vi "Realsense Cam Color Stream Start.vi"(8 "error in (no error)":errorcluster, 11 "Realsense Cam in":refnum<class "Realsense Cam.lvclass">) -> (0 "error out":errorcluster, 3 "Realsense Cam out":refnum<class "Realsense Cam.lvclass">)   [LabVIEW 2018]
uses:
  Realsense Cam.lvclass
  Private/Stream Types Enum STYP.ctl
  Private/Stream STYP.ctl
  Private/Activated Stream STYP.ctl
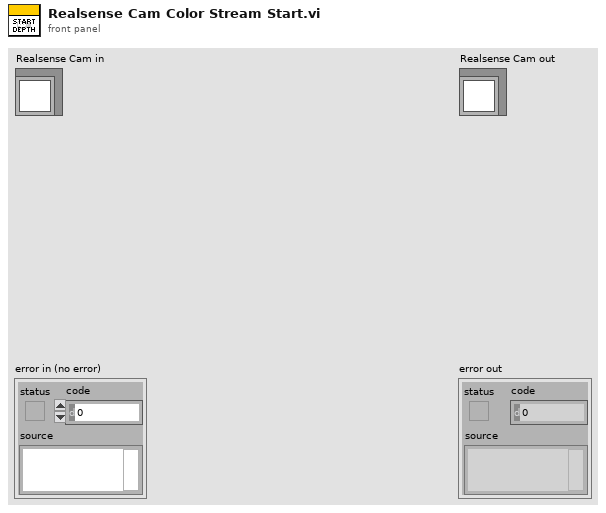
[diagram p1: front panel]
types:
  T1 = typedef "Realsense Cam.lvclass/Activated Stream STYP.ctl" = cluster{"Stream Type":T2, "Resolution":u16, "Profile Handle":u64, "Stream":T3}
  T2 = typedef "Realsense Cam.lvclass/Stream Types Enum STYP.ctl" = enum16{"Depth", "Left IR", "Right IR", "Color", "RGB Ext.", "Left IR Unrectified", "Right IR Unrectified"}
  T3 = typedef "Realsense Cam.lvclass/Stream STYP.ctl" = cluster{"Strings":string[], "Intrinsics":cluster{"width":i32, "height":i32, "fps":i32, "Profile":u64, "ppx":sgl, "ppy":sgl, "fx":sgl, "fy":sgl, "model":u32}[]}
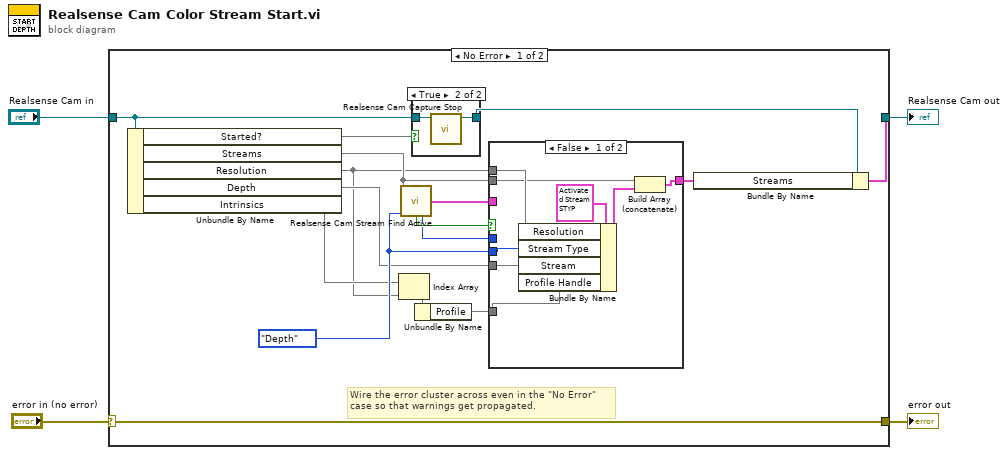
[diagram p0: block diagram]
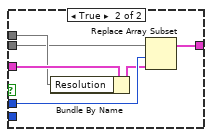
[diagram p2: hidden frame]
diagram:
  n1 = case shown="No Error" "error in (no error)" {
    selector: "error in (no error)" -> [w20 w39]
    tunnel: [w20 w39] -> w3
    tunnel: [w5 w38] -> w1
    tunnel: "Realsense Cam in" -> [w19 w38]
    frame No Error {
      w13 = Stream_Types_Enum_STYP."Depth" ("Stream Types")
      # "Wire the error cluster across even in the \"No Error\"\ncase so that warnings get propagated."
      n2 = Unbundle By Name(w19) -> ("Started?"=w18, "Streams"=w14, "Resolution"=w10, "Depth"=w12, "Intrinsics"=w11)
      n3 = Index Array(array=w11, index=w10) -> (element=w9)
      n4 = call "Realsense Cam Stream Find Active.vi"("Streams"=w14, "Stream Types"=w13) -> ("Activated Stream"=w15:T1, "Found?"=w17:bool, "Index"=w16:i32)  [unwired: 11 in]
      n5 = case shown="True" w18 {
        tunnel: w19 -> [w35 w37]
        tunnel: [w35 w36] -> w7
        frame False {
        }
        frame True {
          n6 = call-dynamic "Realsense Cam Capture Stop.vi"("Realsense Cam in"=w37) -> ("Realsense Cam out"=w36:refnum<class "Realsense Cam.lvclass">)  [unwired: 8 in, 2 out]
        }
      }
      n7 = Unbundle By Name(w9) -> ("Profile"=w8)
      n8 = case shown="False" w17 {
        tunnel: w16 -> [_ w31]
        tunnel: w15 -> [_ w34]
        tunnel: w10 -> [w24 w33]
        tunnel: w14 -> [w23 w32]
        tunnel: w13 -> [w25 _]
        tunnel: [w21 w29] -> w6
        tunnel: w12 -> [w26 _]
        tunnel: w8 -> [w27 _]
        frame False {
          n9 = Bundle By Name(cluster=T1 {"Stream Type"=enum."Color", "Resolution"=17, "Profile Handle"=0, "Stream"={"Strings"=["424 x 240 @6fps", "424 x 240 @15fps", "424 x 240 @30fps", "424 x 240 @60fps", "424 x 240 @90fps", "480 x 270 @6fps", "480 x 270 @15fps", "480 x 270 @30fps", "480 x 270 @60fps", "480 x 270 @90fps", "640 x 360 @6fps", "640 x 360 @15fps", "640 x 360 @30fps", "640 x 360 @60fps", "640 x 360 @90fps", "640 x 480 @6fps", "640 x 480 @15fps", "640 x 480 @30fps", "640 x 480 @60fps", "640 x 480 @90fps", "848 x 480 @6fps", "848 x 480 @15fps", "848 x 480 @30fps", "848 x 480 @60fps", "848 x 480 @90fps", "1280 x 720 @6fps", "1280 x 720 @15fps", "1280 x 720 @30fps", "1920 x 1080 @15fps", "1920 x 1080 @25fps"], "Intrinsics"=[{"width"=424, "height"=240, "fps"=6, "Profile"=521311384, "ppx"=210.19093, "ppy"=123.56658, "fx"=317.53546, "fy"=317.53546, "model"=4}, {"width"=424, "height"=240, "fps"=15, "Profile"=521310104, "ppx"=210.19093, "ppy"=123.56658, "fx"=317.53546, "fy"=317.53546, "model"=4}, {"width"=424, "height"=240, "fps"=30, "Profile"=521314712, "ppx"=210.19093, "ppy"=123.56658, "fx"=317.53546, "fy"=317.53546, "model"=4}, {"width"=424, "height"=240, "fps"=60, "Profile"=521313688, "ppx"=210.19093, "ppy"=123.56658, "fx"=317.53546, "fy"=317.53546, "model"=4}, {"width"=424, "height"=240, "fps"=90, "Profile"=521315736, "ppx"=210.19093, "ppy"=123.56658, "fx"=317.53546, "fy"=317.53546, "model"=4}, {"width"=480, "height"=270, "fps"=6, "Profile"=521314968, "ppx"=237.96481, "ppy"=139.0124, "fx"=357.2274, "fy"=357.2274, "model"=4}, {"width"=480, "height"=270, "fps"=15, "Profile"=521318808, "ppx"=237.96481, "ppy"=139.0124, "fx"=357.2274, "fy"=357.2274, "model"=4}, {"width"=480, "height"=270, "fps"=30, "Profile"=521316504, "ppx"=237.96481, "ppy"=139.0124, "fx"=357.2274, "fy"=357.2274, "model"=4}, {"width"=480, "height"=270, "fps"=60, "Profile"=521322904, "ppx"=237.96481, "ppy"=139.0124, "fx"=357.2274, "fy"=357.2274, "model"=4}, {"width"=480, "height"=270, "fps"=90, "Profile"=521312152, "ppx"=237.96481, "ppy"=139.0124, "fx"=357.2274, "fy"=357.2274, "model"=4}, {"width"=640, "height"=360, "fps"=6, "Profile"=521314200, "ppx"=317.2864, "ppy"=185.34987, "fx"=476.3032, "fy"=476.3032, "model"=4}, {"width"=640, "height"=360, "fps"=15, "Profile"=521319320, "ppx"=317.2864, "ppy"=185.34987, "fx"=476.3032, "fy"=476.3032, "model"=4}, {"width"=640, "height"=360, "fps"=30, "Profile"=521319064, "ppx"=317.2864, "ppy"=185.34987, "fx"=476.3032, "fy"=476.3032, "model"=4}, {"width"=640, "height"=360, "fps"=60, "Profile"=521321112, "ppx"=317.2864, "ppy"=185.34987, "fx"=476.3032, "fy"=476.3032, "model"=4}, {"width"=640, "height"=360, "fps"=90, "Profile"=521318296, "ppx"=317.2864, "ppy"=185.34987, "fx"=476.3032, "fy"=476.3032, "model"=4}, {"width"=640, "height"=480, "fps"=6, "Profile"=521313176, "ppx"=316.38187, "ppy"=247.13316, "fx"=635.0709, "fy"=635.0709, "model"=4}, {"width"=640, "height"=480, "fps"=15, "Profile"=521321368, "ppx"=316.38187, "ppy"=247.13316, "fx"=635.0709, "fy"=635.0709, "model"=4}, {"width"=640, "height"=480, "fps"=30, "Profile"=521309592, "ppx"=316.38187, "ppy"=247.13316, "fx"=635.0709, "fy"=635.0709, "model"=4}, {"width"=640, "height"=480, "fps"=60, "Profile"=521320088, "ppx"=316.38187, "ppy"=247.13316, "fx"=635.0709, "fy"=635.0709, "model"=4}, {"width"=640, "height"=480, "fps"=90, "Profile"=521322648, "ppx"=316.38187, "ppy"=247.13316, "fx"=635.0709, "fy"=635.0709, "model"=4}, {"width"=848, "height"=480, "fps"=6, "Profile"=521315992, "ppx"=420.38187, "ppy"=247.13316, "fx"=635.0709, "fy"=635.0709, "model"=4}, {"width"=848, "height"=480, "fps"=15, "Profile"=521317272, "ppx"=420.38187, "ppy"=247.13316, "fx"=635.0709, "fy"=635.0709, "model"=4}, {"width"=848, "height"=480, "fps"=30, "Profile"=521310616, "ppx"=420.38187, "ppy"=247.13316, "fx"=635.0709, "fy"=635.0709, "model"=4}, {"width"=848, "height"=480, "fps"=60, "Profile"=521310360, "ppx"=420.38187, "ppy"=247.13316, "fx"=635.0709, "fy"=635.0709, "model"=4}, {"width"=848, "height"=480, "fps"=90, "Profile"=521306776, "ppx"=420.38187, "ppy"=247.13316, "fx"=635.0709, "fy"=635.0709, "model"=4}, {"width"=1280, "height"=720, "fps"=6, "Profile"=521320600, "ppx"=634.5728, "ppy"=370.69974, "fx"=952.6064, "fy"=952.6064, "model"=4}, {"width"=1280, "height"=720, "fps"=15, "Profile"=521310872, "ppx"=634.5728, "ppy"=370.69974, "fx"=952.6064, "fy"=952.6064, "model"=4}, {"width"=1280, "height"=720, "fps"=30, "Profile"=521320344, "ppx"=634.5728, "ppy"=370.69974, "fx"=952.6064, "fy"=952.6064, "model"=4}, {"width"=1920, "height"=1080, "fps"=15, "Profile"=521627576, "ppx"=951.85925, "ppy"=556.0496, "fx"=1428.9095, "fy"=1428.9095, "model"=4}, {"width"=1920, "height"=1080, "fps"=25, "Profile"=521617080, "ppx"=951.85925, "ppy"=556.0496, "fx"=1428.9095, "fy"=1428.9095, "model"=4}]}} ("Activated Stream"), "Resolution"=w24, "Stream Type"=w25, "Stream"=w26, "Profile Handle"=w27) -> (w22:T1)
          n10 = Build Array (concatenate)(w23, w22) -> (w21:T1[])
        }
        frame True {
          n11 = Bundle By Name(cluster=w34, "Resolution"=w33) -> (w30:T1)
          n12 = Replace Array Subset(array=w32, new element=w30, index=w31) -> (w29:T1[])
        }
      }
      n13 = Bundle By Name(cluster=w7, "Streams"=w6) -> (w5:cluster{})
    }
    frame Error {
    }
  }
  "error out" <- w3
  "Realsense Cam out" <- w1
